vi "GoBang_WinSituation.vi"(0 "GameBoard":u8[][](array[numeric])) -> (1 "White won":bool, 2 "Black won":bool, 3 "Game over":bool)   [LabVIEW 2014, in "GoBang.lvlib"]
uses:
  GoBang.lvlib
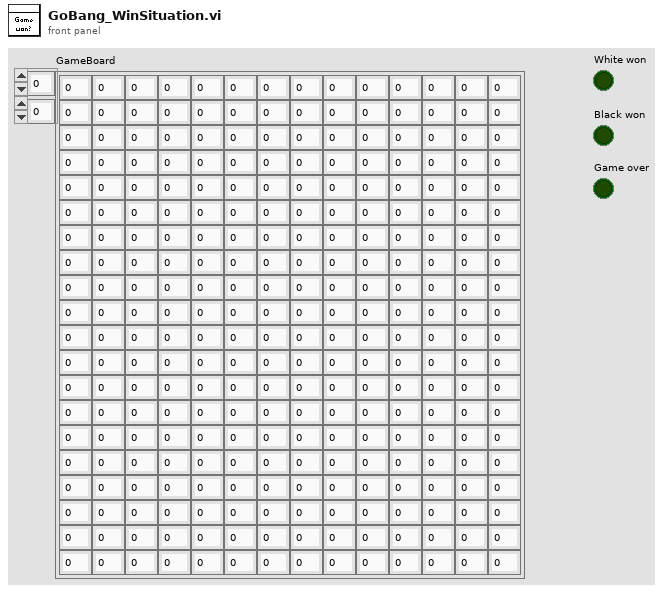
[diagram p1: front panel]
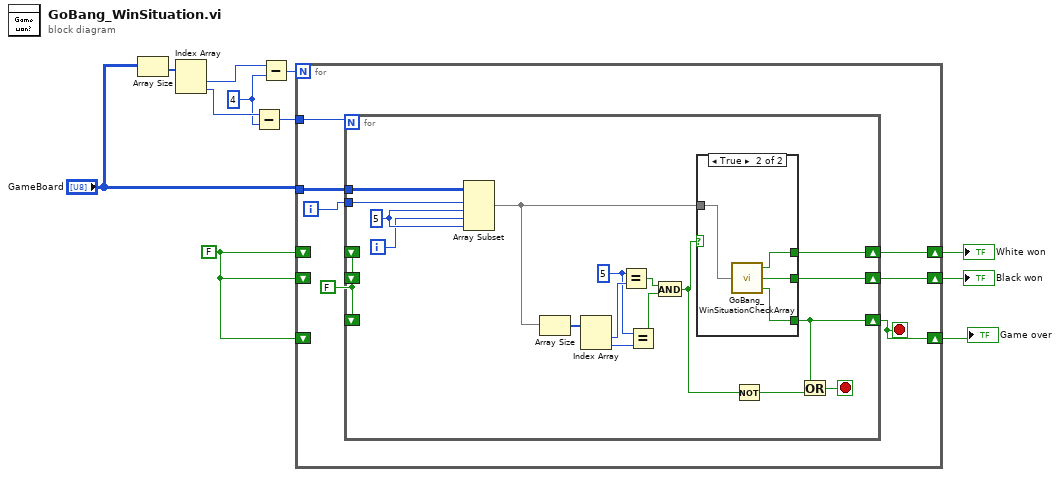
[diagram p0: block diagram]
diagram:
  w1 = 4 ("y")
  w8 = FALSE
  n1 = Array Size(array="GameBoard") -> (size(s)=w6:i32[])
  n2 = Index Array(array=w6) -> (element #1=w5:i32, element #2=w3:i32)  [unwired: 2 in]
  n3 = Subtract(x=w3, y=w1) -> (x-y=w2:i32)
  n4 = Subtract(x=w5, y=w1) -> (x-y=w4:i32)
  n5 = for {
    N: w4 -> [_]
    tunnel: "GameBoard" -> [w18]
    shift-right: [w16] -> w11
    shift-left: w8 -> [_]
    shift-right: [w15] -> w10
    shift-left: w8 -> [_]
    shift-right: [w14] -> w9
    shift-left: w8 -> [_]
    tunnel: w2 -> [w12]
    i -> [w17]
    stop <- w14 stop-if-true
    w13 = FALSE
    n6 = for {
      N: w12 -> [_]
      tunnel: w18 -> [w35]
      tunnel: w17 -> [w32]
      shift-right: [w26] -> w14
      shift-left: w13 -> [_]
      shift-right: [w29] -> w16
      shift-left: w13 -> [_]
      shift-right: [w28] -> w15
      shift-left: w13 -> [_]
      i -> [w33]
      stop <- w27 stop-if-true
      w23 = 5 ("x")
      w34 = 5 ("row N")
      n7 = Array Subset(array=w35, index (row)=w32, length (row)=w34, index (col)=w33, length (col)=w34) -> (w30:u8[][])
      n8 = Array Size(array=w30) -> (size(s)=w31:i32[])
      n9 = Index Array(array=w31) -> (element #1=w25:i32, element #2=w24:i32)  [unwired: 2 in]
      n10 = Equal?(x=w23, y=w25) -> (x = y?=w22:bool)
      n11 = Equal?(x=w23, y=w24) -> (x = y?=w21:bool)
      n12 = And(x=w22, y=w21) -> (x .and. y?=w20:bool)
      n13 = case shown="True" w20 {
        tunnel: w30 -> [_ w39]
        tunnel: [_ w38] -> w29
        tunnel: [_ w37] -> w28
        tunnel: [_ w36] -> w26
        frame False {
        }
        frame True {
          n14 = call "GoBang_WinSituationCheckArray.vi"("5x5 array"=w39) -> ("white won"=w38:bool, "black won"=w37:bool, "game over"=w36:bool)
        }
      }
      n15 = Not(x=w20) -> (.not. x?=w19:bool)
      n16 = Or(x=w26, y=w19) -> (x .or. y?=w27:bool)
    }
  }
  "White won" <- w11
  "Black won" <- w10
  "Game over" <- w9
